vi "Power Scan.vi"(8 "# Steps":dbl, 9 "Max (mW)":dbl, 10 "Min (mW)":dbl, 11 "file path (dialog if empty)":path) -> (3 "XY Graph":cluster{"Y":dbl[], "Y":dbl[]}[](graph))   [LabVIEW 2012]
uses:
  <vilib>/Utility/file.llb/Write To Spreadsheet File (DBL).vi
  F:/Users/Ouyang Group/Documents/Colton LabView code/Instruments/Laser power controller/BEOC LPC/BEOC LPC.lvlib
panel:
  in  "stop":bool
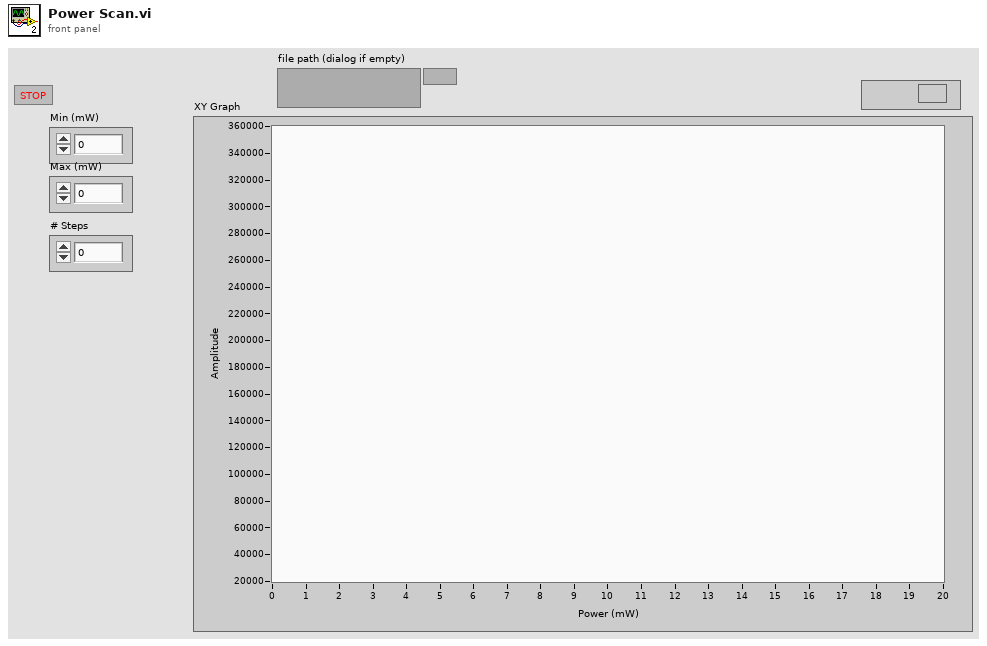
[diagram p1: front panel]
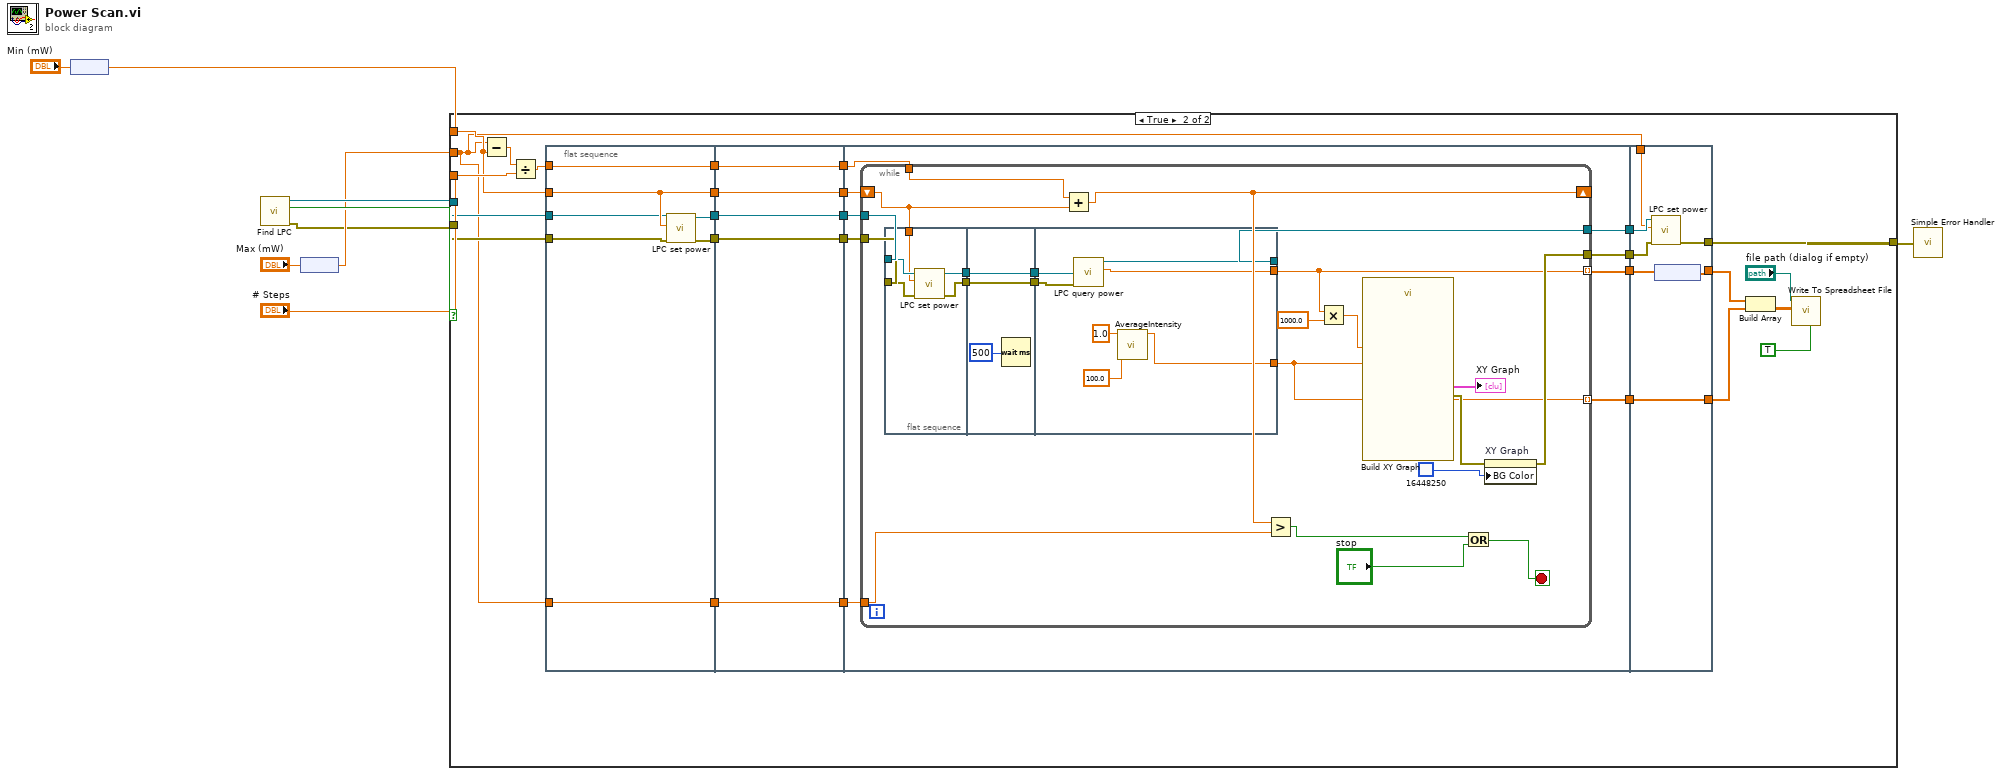
[diagram p0: block diagram]
diagram:
  n1 = node("Min (mW)") -> (w6:dbl[unit])
  n2 = call "Find LPC.vi"() -> ("error out"=w2:errorcluster, "LPC found?"=w9:bool, "VISA resource name out"=w8:refnum<visa-resource-name>)  [unwired: 9 in]
  n3 = node("Max (mW)") -> (w4:dbl[unit])
  n4 = case shown="True" w9 {
    tunnel: w8 -> [_ w37]
    tunnel: w2 -> [w10 w36]
    tunnel: w6 -> [_ w20]
    tunnel: w4 -> [_ w11]
    tunnel: "# Steps" -> [_ w33]
    tunnel: [w10 w19] -> w1
    frame False {
    }
    frame True {
      n5 = Subtract(x=w11, y=w20) -> (x-y=w35:dbl[unit])
      n6 = Divide(x=w35, y=w33) -> (x/y=w34:dbl[unit])
      n7 = flat-sequence {
        tunnel: w11 -> [w43]
        tunnel: w34 -> [w44]
        tunnel: w20 -> [w40]
        tunnel: w36 -> [w38]
        tunnel: w37 -> [w39]
        tunnel: [w41] -> w32
        tunnel: [w42] -> w30
        tunnel: [w40] -> w28
        tunnel: [w44] -> w26
        tunnel: [w43] -> w24
        tunnel: w32 -> [w49]
        tunnel: [w49] -> w31
        tunnel: w30 -> [w48]
        tunnel: [w48] -> w29
        tunnel: w28 -> [w47]
        tunnel: [w47] -> w27
        tunnel: w26 -> [w46]
        tunnel: [w46] -> w25
        tunnel: w24 -> [w45]
        tunnel: [w45] -> w23
        tunnel: w31 -> [w58]
        tunnel: w29 -> [w57]
        tunnel: w27 -> [w56]
        tunnel: w25 -> [w55]
        tunnel: w23 -> [w54]
        tunnel: [w53] -> w22
        tunnel: [w52] -> w21
        tunnel: [w51] -> w18
        tunnel: [w50] -> w17
        tunnel: w22 -> [w102]
        tunnel: w21 -> [w101]
        tunnel: w11 -> [w100]
        tunnel: [w99] -> w19
        tunnel: [w96] -> w16
        tunnel: w18 -> [w97]
        tunnel: [w98] -> w15
        tunnel: w17 -> [w98]
        frame #0 {
          n8 = call "LPC set power.vi"("error in (no error)"=w38, "power"=w40, "VISA resource name"=w39) -> ("error out"=w42:errorcluster, "VISA resource name out"=w41:refnum<visa-resource-name>)  [unwired: 7 in]
        }
        frame #1 {
        }
        frame #2 {
          n9 = while {
            shift-right: [w77] -> _
            shift-left: w56 -> [w72]
            tunnel: w58 -> [w80]
            tunnel: w57 -> [w79]
            tunnel: w55 -> [w78]
            tunnel: w54 -> [w76]
            tunnel: [w70] -> w53
            tunnel: [w67] -> w52
            tunnel: [w60] -> w51 mode=indexing
            tunnel: [w59] -> w50 mode=indexing
            stop <- w73 stop-if-true
            n10 = flat-sequence {
              tunnel: w80 -> [w85]
              tunnel: w79 -> [w84]
              tunnel: [w83] -> w64
              tunnel: w72 -> [w82]
              tunnel: [w81] -> w62
              tunnel: w64 -> [w88]
              tunnel: [w88] -> w63
              tunnel: w62 -> [w87]
              tunnel: [w87] -> w61
              tunnel: w63 -> [w94]
              tunnel: w61 -> [w95]
              tunnel: [w93] -> w70
              tunnel: [w92] -> w60
              tunnel: [w91] -> w59
              frame #0 {
                n11 = call "LPC set power.vi"("error in (no error)"=w84, "power"=w82, "VISA resource name"=w85) -> ("error out"=w83:errorcluster, "VISA resource name out"=w81:refnum<visa-resource-name>)  [unwired: 7 in]
              }
              frame #1 {
                n12 = Wait (ms)(milliseconds to wait=u32 500) -> ()  [unwired: 1 out]
              }
              frame #2 {
                n13 = call "LPC query power.vi"("error in (no error)"=w94, "VISA resource name"=w95) -> ("power"=w92:dbl[unit], "VISA resource name out"=w93:refnum<visa-resource-name>)  [unwired: 7 in, 1 out]
                n14 = call "AverageIntensity.vi"("rate (Hz)"=100.0, "Time Target (s)"=1.0) -> ("Average intensity (cts/s)"=w91:dbl)  [unwired: 8 in, 1 out]
              }
            }
            n15 = Add(x=w78, y=w72) -> (x+y=w77:dbl[unit])
            n16 = Greater?(x=w77, y=w76) -> (0:w74:bool)
            n17 = Multiply(x=w60, y=dbl[unit] 1000.0) -> (x*y=w65:dbl[unit])
            n18 = call "Build XY Graph"("Y Input"=w59, "X Input"=w65) -> ("error out"=w68:errorcluster, "XY Graph"=→"XY Graph":cluster{"Y":dbl[], "Y":dbl[]}[])  [unwired: 3 in, 5 out]
            n19 = Or(x=w74, y="stop") -> (x .or. y?=w73:bool)
            n20 = property on="XY Graph" class="XYGraph (strict)"(error in=w68, "BG Color"=u32 16448250) -> (error out=w67:errorcluster)  [unwired: 1 in, 1 out]
          }
        }
        frame #3 {
          n21 = call "LPC set power.vi"("error in (no error)"=w101, "power"=w100, "VISA resource name"=w102) -> ("error out"=w99:errorcluster)  [unwired: 7 in, 1 out]
          n22 = node(w97) -> (w96:dbl[])
        }
      }
      n23 = Build Array(w16, w15) -> (w14:dbl[][])
      n24 = call-poly <vilib>:"Write To Spreadsheet File.vi"("transpose? (no:F)"=TRUE, "2D data"=w14, "file path (dialog if empty)"="file path (dialog if empty)") -> ()  [unwired: 5 in, 1 out]
    }
  }
  n25 = call <vilib>:"Simple Error Handler.vi"("error in (no error)"=w1) -> ()  [unwired: 4 in, 5 out]
